vi "Create - DML.vi"(8 "error in (no error)":errorcluster) -> (0 "error out":errorcluster, 3 "DriveMotors out":refnum<class "DriveMotors.lvclass">)   [LabVIEW 2013]
uses:
  Systems/DriveMotors/DriveMotors.lvclass
  <vilib>/Rock Robotics/SystemInterfaces/DIO/FPGA_DIOChannel.ctl
  <vilib>/Rock Robotics/WPI/Encoder/WPI_EncoderType.ctl
  <vilib>/Utility/config.llb/Read Key (Boolean).vi
  <vilib>/Utility/config.llb/NI_LVConfig.lvlib
panel:
  in  "Encoder Number Samples to Average":u8=4 min=1 max=128
  in  "Encoder Minimum Rate":dbl=100.0
  in  "Encoder Invert Direction":bool
  in  "Enum":T1=enum."4x"
  in  "B DIOChannel":T2=enum."DIO 7"
  in  "A DIOChannel":T2=enum."DIO 6"
  in  "Sync Group":u8=2 format="%08b"
  in  "Motor3CAN":u8=16
  in  "Motor2CAN":u8=15
  in  "Motor1CAN":u8=14
  in  "Invert Motors":bool
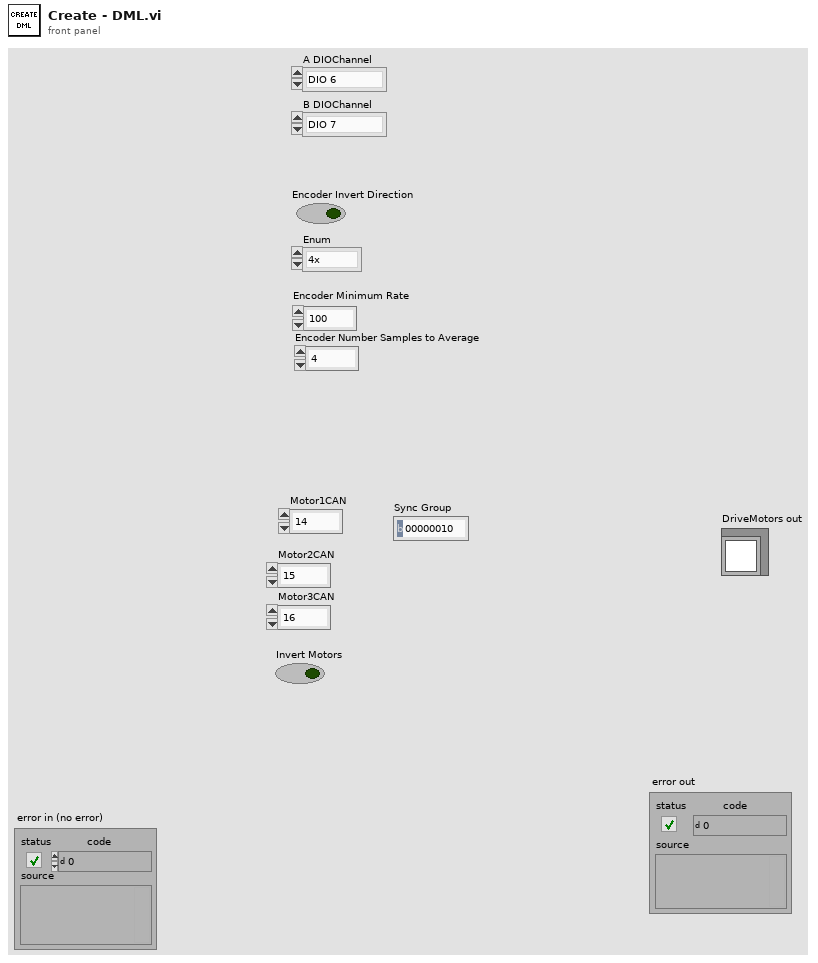
[diagram p1: front panel]
types:
  T1 = typedef "WPI_EncoderType.ctl" = enum16{"1x", "2x", "4x"}
  T2 = typedef "FPGA_DIOChannel.ctl" = enum8{"DIO 1", "DIO 2", "DIO 3", "DIO 4", "DIO 5", "DIO 6", "DIO 7", "DIO 8", "DIO 9", "DIO 10", "DIO 11", "DIO 12", "DIO 13", "DIO 14", "Invalid"}
  T3 = typedef "NI_LVConfig.lvlib/Config Data RefNum.ctl" = refnum<k1>
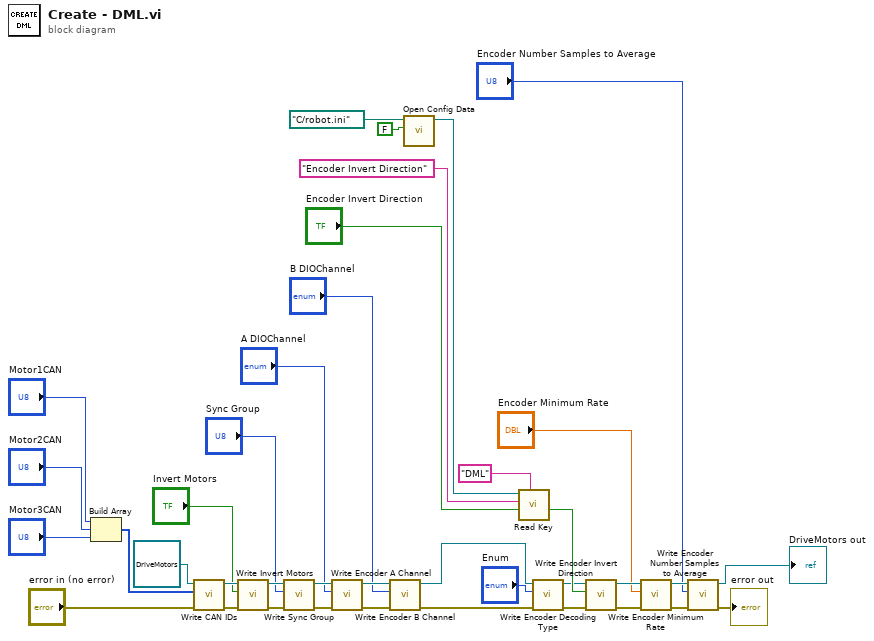
[diagram p0: block diagram]
diagram:
  n1 = Build Array("Motor1CAN", "Motor2CAN", "Motor3CAN") -> (w34:u8[])
  n2 = call-dynamic "Write CAN IDs.vi"("error in (no error)"="error in (no error)", "CAN IDs"=w34, "DriveMotors in"=refnum<class "DriveMotors.lvclass"> refnum ("DriveMotors.lvclass")) -> ("error out"=w30:errorcluster, "DriveMotors out"=w33:refnum<class "DriveMotors.lvclass">)  [unwired: 7 in]
  n3 = call-dynamic "Write Invert Motors.vi"("error in (no error)"=w30, "Invert Motors"="Invert Motors", "DriveMotors in"=w33) -> ("error out"=w29:errorcluster, "DriveMotors out"=w28:refnum<class "DriveMotors.lvclass">)  [unwired: 7 in]
  n4 = call-dynamic "Write Sync Group.vi"("error in (no error)"=w29, "Sync Group"="Sync Group", "DriveMotors in"=w28) -> ("error out"=w14:errorcluster, "DriveMotors out"=w13:refnum<class "DriveMotors.lvclass">)  [unwired: 7 in]
  n5 = call-dynamic "Write Encoder A Channel.vi"("error in (no error)"=w14, "A DIOChannel"="A DIOChannel", "DriveMotors in"=w13) -> ("error out"=w24:errorcluster, "DriveMotors out"=w26:refnum<class "DriveMotors.lvclass">)  [unwired: 7 in]
  n6 = call-dynamic "Write Encoder B Channel.vi"("error in (no error)"=w24, "B DIOChannel"="B DIOChannel", "DriveMotors in"=w26) -> ("error out"=w23:errorcluster, "DriveMotors out"=w25:refnum<class "DriveMotors.lvclass">)  [unwired: 7 in]
  n7 = call <vilib>:"Open Config Data.vi"("create file if necessary (T)"=FALSE, "configuration file path"=path "C:/robot.ini") -> ("refnum"=w5:T3)  [unwired: 7 in, 2 out]
  n8 = call-poly <vilib>:"Read Key.vi"("section"="DML", "default value"="Encoder Invert Direction", "key"="Encoder Invert Direction", "refnum"=w5) -> ("value"=w8:bool)  [unwired: 4 in, 3 out]
  n9 = call-dynamic "Write Encoder Decoding Type.vi"("error in (no error)"=w23, "Enum"="Enum", "DriveMotors in"=w25) -> ("error out"=w2:errorcluster, "DriveMotors out"=w4:refnum<class "DriveMotors.lvclass">)  [unwired: 7 in]
  n10 = call-dynamic "Write Encoder Invert Direction.vi"("error in (no error)"=w2, "Encoder Invert Direction"=w8, "DriveMotors in"=w4) -> ("error out"=w17:errorcluster, "DriveMotors out"=w18:refnum<class "DriveMotors.lvclass">)  [unwired: 7 in]
  n11 = call-dynamic "Write Encoder Minimum Rate.vi"("error in (no error)"=w17, "Encoder Minimum Rate"="Encoder Minimum Rate", "DriveMotors in"=w18) -> ("error out"=w20:errorcluster, "DriveMotors out"=w19:refnum<class "DriveMotors.lvclass">)  [unwired: 7 in]
  n12 = call-dynamic "Write Encoder Number Samples to Average.vi"("error in (no error)"=w20, "Encoder Number Samples to Average"="Encoder Number Samples to Average", "DriveMotors in"=w19) -> ("error out"=→"error out":errorcluster, "DriveMotors out"=→"DriveMotors out":refnum<class "DriveMotors.lvclass">)  [unwired: 7 in]
